vi "Get Dependency Projects.vi"(8 "error in (no error)":errorcluster, 11 "PackageAbstract in":refnum<class "PackageAbstract.lvclass">) -> (0 "error out":errorcluster, 2 "Dependencies":refnum<class "Package.lvclass">[](array[class]), 3 "PackageAbstract out":refnum<class "PackageAbstract.lvclass">)   [LabVIEW 2020, in "GPack.lvlib" / "PackageAbstract.lvclass"]
uses:
  PackageAbstract.lvclass
  Package/Package.lvclass
  PackageAbstract.lvclass/PackageAbstract.ctl
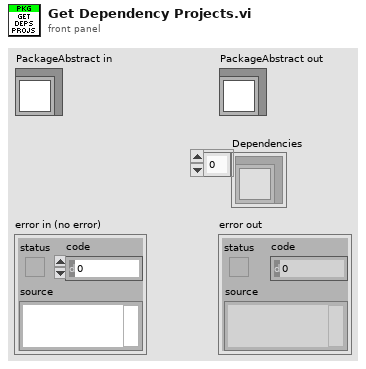
[diagram p1: front panel]
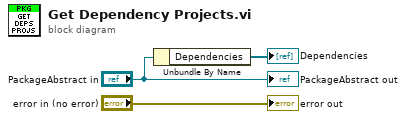
[diagram p0: block diagram]
diagram:
  n1 = Unbundle By Name("PackageAbstract in") -> ("Dependencies"=→"Dependencies":refnum<class "Package.lvclass">[])
  "error out" <- "error in (no error)"
  "PackageAbstract out" <- "PackageAbstract in"
